vi "Write Number of subscriptions.vi"(8 "error in (no error)":errorcluster, 10 "Number of subscriptions":u64, 11 "SubscriptionDetailsParent in":refnum<class "SubscriptionDetailsParent.lvclass">) -> (0 "error out":errorcluster, 3 "SubscriptionDetailsParent out":refnum<class "SubscriptionDetailsParent.lvclass">)   [LabVIEW 2020, in "wamplv.lvlib" / "SubscriptionDetailsParent.lvclass"]
uses:
  SubscriptionDetailsParent.lvclass
  SubscriptionDetailsParent.lvclass/SubscriptionDetailsParent.ctl
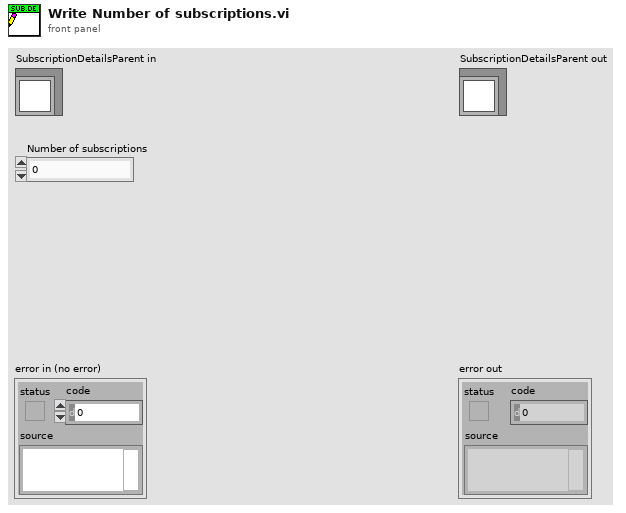
[diagram p1: front panel]
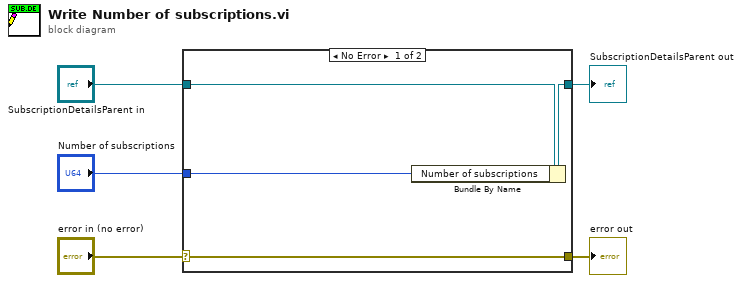
[diagram p0: block diagram]
diagram:
  n1 = case shown="No Error" "error in (no error)" {
    selector: "error in (no error)" -> [w9 w10]
    tunnel: [w9 w10] -> w4
    tunnel: [w7 w11] -> w2
    tunnel: "SubscriptionDetailsParent in" -> [w8 w11]
    tunnel: "Number of subscriptions" -> [w6 _]
    frame No Error {
      n2 = Bundle By Name(cluster=w8, "Number of subscriptions"=w6) -> (w7:refnum<class "SubscriptionDetailsParent.lvclass">)
    }
    frame Error {
    }
  }
  "error out" <- w4
  "SubscriptionDetailsParent out" <- w2
